vi "Get Polygon Marker.vi"(8 "Error In":errorcluster, 11 "Point":refnum<k24>) -> (0 "error out":errorcluster, 3 "new reference":refnum<k24>)   [LabVIEW 2014]
uses:
  C:/Robotic Systems/Products/AgFalcon/Software/Ground Station/Data/Mapping DLL/GMap.NET.WindowsForms.dll
  Data/Mapping DLL/GMap.NET.WindowsForms.dll
  C:/Robotic Systems/Products/AgFalcon/Software/Ground Station/Data/Mapping DLL/GMap.NET.Core.dll
  Data/Mapping DLL/GMap.NET.Core.dll
  System.Drawing
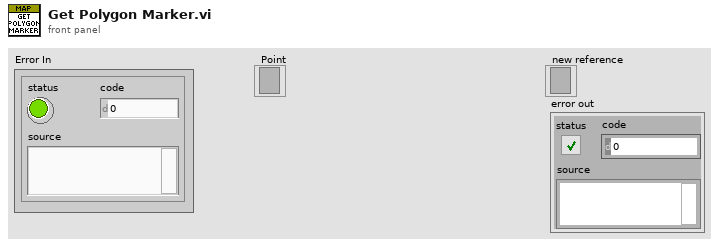
[diagram p1: front panel]
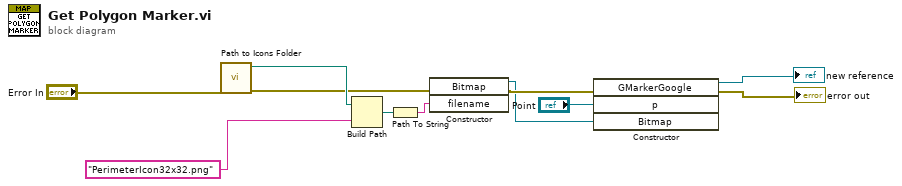
[diagram p0: block diagram]
diagram:
  n1 = call "Path to Icons Folder.vi"("Error In"="Error In") -> ("Error Out"=w8:errorcluster, "Path to Icons Folder"=w10:path)  [unwired: 9 in]
  n2 = Build Path(base path=w10, name or relative path="PerimeterIcon32x32.png" ("Plant Icon")) -> (appended path=w9:path)
  n3 = Path To String(path=w9) -> (string=w11:string)
  n4 = constructor class="Bitmap"(error in=w8, "filename"=w11) -> (reference out=w6:refnum<k24>, error out=w7:errorcluster)  [unwired: 2 in, 2 out]
  n5 = constructor class="GMarkerGoogle"(error in=w7, "p"="Point", "Bitmap"=w6) -> (reference out=→"new reference":refnum<k24>, error out=→"error out":errorcluster)  [unwired: 2 in, 3 out]
